vi "NS Reader.vi"(8 "error in":errorcluster, 10 "notifier in":refnum<notifier>, 11 "Message Queues in":T1) -> (0 "error out":errorcluster, 2 "Available Elements for Reading":i32)   [LabVIEW 2022 SP3]
uses:
  UI Message handler/Message Queue/All Message Queues.ctl
  UI Message handler/Message Queue/Message Cluster.ctl
  Controls/Notifier data ctl.ctl
  Globals/Phase III Globals.vi
  UI Message handler/Message Queue/Message Queue.lvlib
  <resource>/objmgr/ni.dex.rc
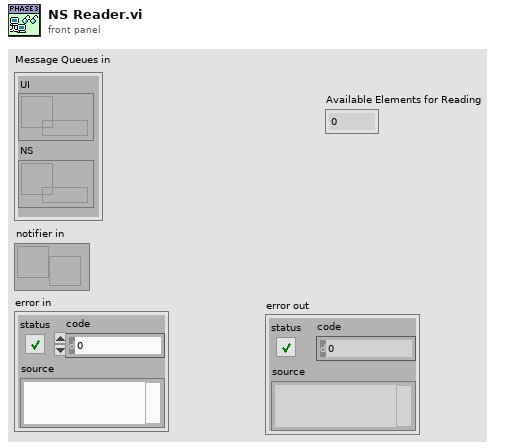
[diagram p1: front panel]
types:
  T1 = typedef "Message Queue.lvlib/All Message Queues.ctl" = cluster{"UI":refnum<queue>, "NS ":refnum<queue>}
  T2 = typedef "NS Data type.ctl" = cluster{string, variant}
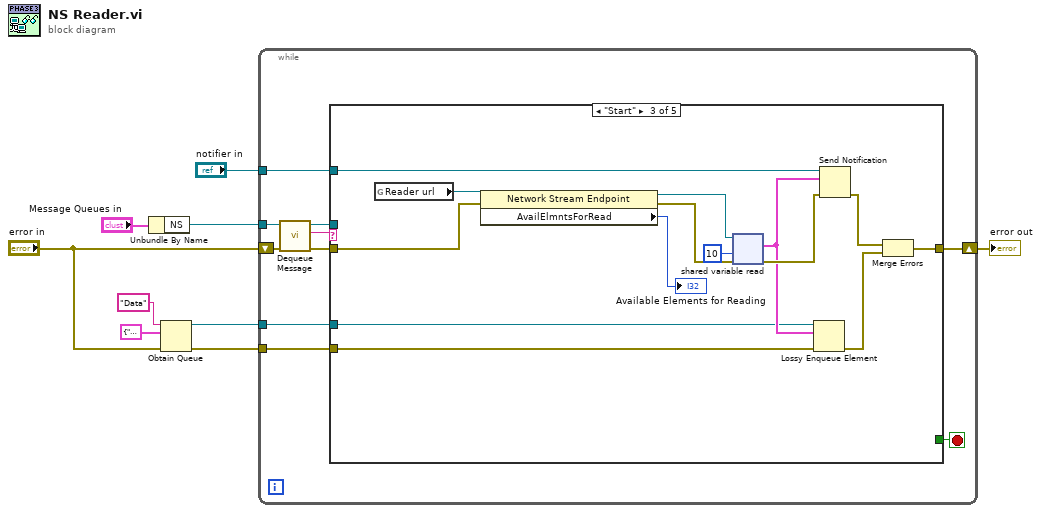
[diagram p0: block diagram]
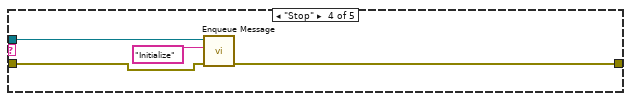
[diagram p4: hidden frame]
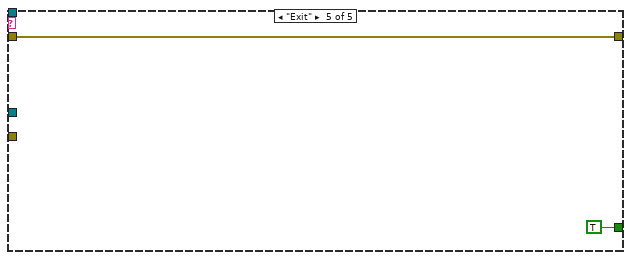
[diagram p5: hidden frame]
diagram:
  n1 = Unbundle By Name("Message Queues in") -> ("NS"=w8:refnum<queue>)
  n2 = Obtain Queue(name (unnamed)="Data", element data type=cluster{string, variant} {"", variant}, error in (no error)="error in") -> (queue out=w3:refnum<queue>, error out=w2:errorcluster)  [unwired: 2 in, 1 out]
  n3 = while {
    tunnel: w8 -> [w16]
    shift-right: [w13] -> w6
    shift-left: "error in" -> [w17]
    tunnel: "notifier in" -> [w12]
    tunnel: w3 -> [w11]
    tunnel: w2 -> [w10]
    stop <- w19 stop-if-true
    n4 = call "Dequeue Message.vi"("error in (no error)"=w17, "Message Queue"=w16) -> ("error out"=w14:errorcluster, "Message"=w18:string, "dup Message Queue"=w15:refnum<queue>)  [unwired: 6 in, 1 out]
    n5 = case shown="\"Start\"" w18 {
      tunnel: [_ _ _ _ TRUE] -> w19
      tunnel: w15 -> [_ _ _ w39 _]
      tunnel: w14 -> [w20 w21 w32 w37 w40]
      tunnel: [w20 w21 w23 w36 w40] -> w13
      tunnel: w12 -> [_ _ w30 _ _]
      tunnel: w11 -> [_ _ w25 _ _]
      tunnel: w10 -> [_ _ w24 _ _]
      frame Default {
      }
      frame "Initialize" {
      }
      frame "Start" {
        n6 = global read "Phase III Globals.vi" "Reader url"() -> (w35:refnum<k21>)
        n7 = property class="Network Stream Endpoint"(reference=w35, error in=w32) -> (reference out=w34:refnum<k21>, error out=w33:errorcluster, "AvailElmntsForRead"=→"Available Elements for Reading":i32)
        n8 = shared-variable-read(w34, w33, 10 ("timeout ms (-1)")) -> (w29:errorcluster, w26:T2)  [unwired: 2 out]
        n9 = Lossy Enqueue Element(queue=w25, element=w26, error in (no error)=w24) -> (error out=w22:errorcluster)  [unwired: 3 out]
        n10 = Send Notification(notification=w26, notifier=w30, error in (no error)=w29) -> (error out=w28:errorcluster)  [unwired: 1 out]
        n11 = Merge Errors(w28, w22) -> (w23:errorcluster)
      }
      frame "Stop" {
        n12 = call "Enqueue Message.vi"("error in (no error)"=w37, "Message"="Initialize", "Message Queue"=w39) -> ("error out"=w36:errorcluster)  [unwired: 7 in, 1 out]
      }
      frame "Exit" {
      }
    }
  }
  "error out" <- w6
